vi "configure.vi"(8 "error in (no error)":errorcluster, 9 "Value":i32, 10 "ILC":refnum<class "ILC.lvclass">, 11 "IConfigureILCStrategy in":refnum<class "IConfigureILCStrategy.lvclass">) -> (0 "error out":errorcluster, 2 "ILC 2":refnum<class "ILC.lvclass">, 3 "IConfigureILCStrategy out":refnum<class "IConfigureILCStrategy.lvclass">)   [LabVIEW 2016, in "IConfigureILCStrategy.lvclass"]
uses:
  IConfigureILCStrategy.lvclass
  Common_ILC/ILC/ILC.lvclass
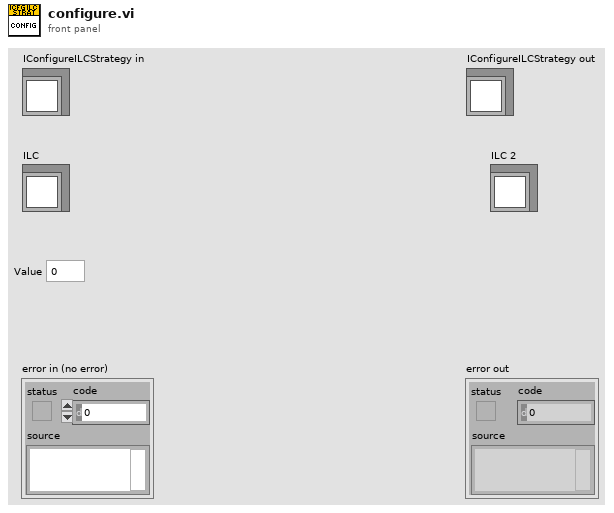
[diagram p1: front panel]
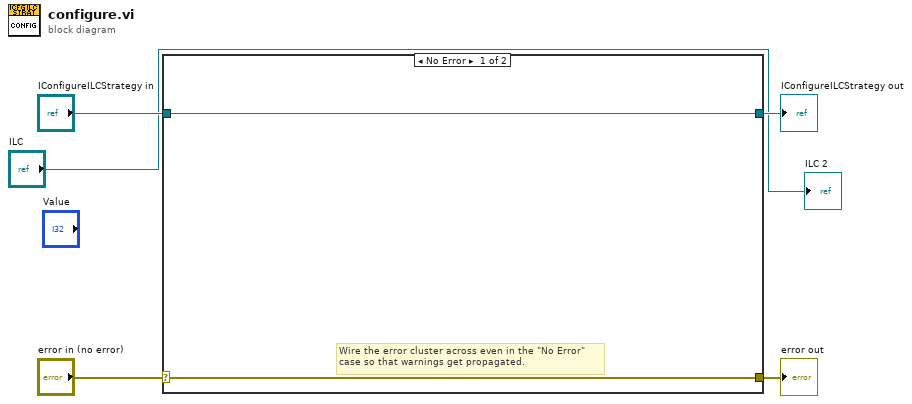
[diagram p0: block diagram]
diagram:
  n1 = case shown="No Error" "error in (no error)" {
    selector: "error in (no error)" -> [w6 w9]
    tunnel: [w6 w9] -> w4
    tunnel: [w7 w8] -> w2
    tunnel: "IConfigureILCStrategy in" -> [w7 w8]
    frame No Error {
      # "Wire the error cluster across even in the \"No Error\"\ncase so that warnings get propagated."
    }
    frame Error {
    }
  }
  "error out" <- w4
  "IConfigureILCStrategy out" <- w2
  "ILC 2" <- "ILC"
